vi "Lex Empty Tag.vi"(8 "Error In":errorcluster) -> (0 "Error Out":errorcluster)   [LabVIEW 2018, in "Tests.lvlib" / "Lexer.lvlib"]
uses:
  Lexer.lvlib
  src/Toolkit/Low-Level/Tokens/EscapedVariable/EscapedVariable.lvclass
  <vilib>/addons/_JKI Toolkits/Caraya/classes/Assert/Assert Equal Type_Variant.vi
  src/Toolkit/Low-Level/Tokens/Keyable/Keyable.lvclass
  src/Toolkit/Low-Level/Lexer/Lexer.lvclass
  <vilib>/addons/_JKI Toolkits/Caraya/classes/Test/Test.lvclass
  <vilib>/addons/_JKI Toolkits/Caraya/classes/Assert/Assert.lvclass
  Tests.lvlib
  src/Toolkit/Low-Level/Tokens/Token/Token.lvclass
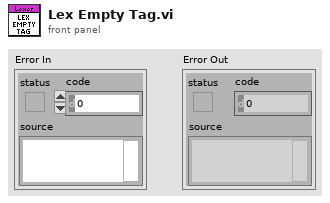
[diagram p1: front panel]
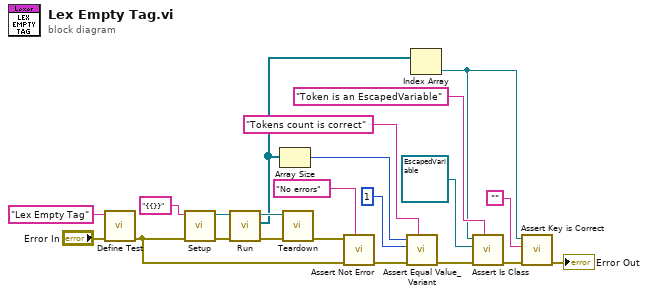
[diagram p0: block diagram]
diagram:
  n1 = call <vilib>:"Define Test.vi"("error in (no error)"="Error In", "Label (VI Title)"="Lex Empty Tag") -> ("error out"=w4:errorcluster)  [unwired: 9 in]
  n2 = call "Setup.vi"("Error In"=w4, "String"="{{}}") -> ("Error Out"=w7:errorcluster, "Lexer"=w8:refnum<class "Lexer.lvclass">)  [unwired: 8 in]
  n3 = call-dynamic "Run.vi"("Error In"=w7, "Lexer In"=w8) -> ("Error Out"=w5:errorcluster, "Tokens"=w1:refnum<class "Token.lvclass">[], "Lexer Out"=w6:refnum<class "Lexer.lvclass">)  [unwired: 7 in]
  n4 = Array Size(array=w1) -> (size(s)=w17:i32)
  n5 = call "Teardown.vi"("Error In"=w5, "Lexer"=w6) -> ("Error Out"=w2:errorcluster)  [unwired: 9 in]
  n6 = call <vilib>:"Assert Not Error.vi"("Label"="No errors", "error in (no error)"=w4, "Not Error?"=w2) -> ("error out"=w19:errorcluster)  [unwired: 8 in]
  n7 = call <vilib>:"Assert Equal Value_Variant.vi"("Label"="Tokens count is correct", "error in (no error)"=w19, "Y"=1 ("size(s)"), "X"=w17) -> ("error out"=w14:errorcluster)  [unwired: 7 in]
  n8 = Index Array(array=w1) -> (element=w9:refnum<class "Token.lvclass">)  [unwired: 1 in]
  n9 = call "Assert Is Class.vi"("Label"="Token is an EscapedVariable", "Error In"=w14, "Expected"=refnum<class "EscapedVariable.lvclass"> refnum ("Mustache.lvlib:Tokens.lvlib:Tag.lvclass"), "Actual"=w9) -> ("Error Out"=w10:errorcluster)  [unwired: 7 in]
  n10 = call "Assert Key is Correct.vi"("Error In"=w10, "Expected"="", "Token"=w9) -> ("Error Out"=→"Error Out":errorcluster)  [unwired: 8 in]
